vi "UI.vi"(8 "error in (no error)":errorcluster, 10 "subPanel":refnum<vi>, 11 "UI in":refnum<class "UI.lvclass">) -> (0 "error out":errorcluster, 3 "UI out":refnum<class "UI.lvclass">)   [LabVIEW 2019, in "UI.lvclass"]
doc: "Opens the UI Session. You need to pass a SubPanel Reference in order to make your embedded VIs show in it. This is the very first fuction you need to call."
uses:
  UI.lvclass
  UI.lvclass/UI.ctl
  setsubPanel.vi
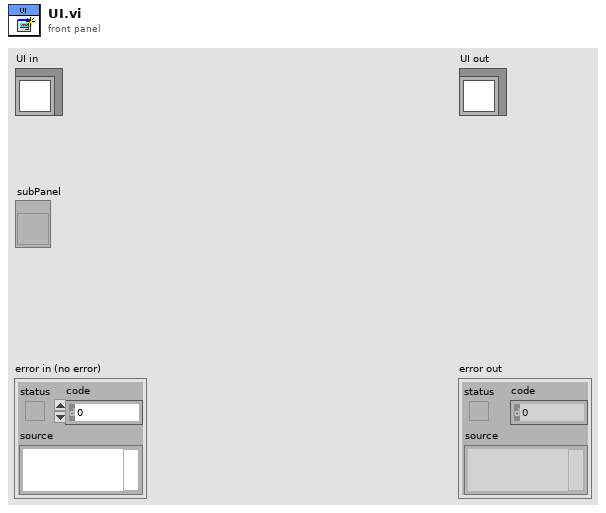
[diagram p1: front panel]
types:
  T1 = enum16{"Create", "Register", "Generate", "Unregister", "Destroy"}
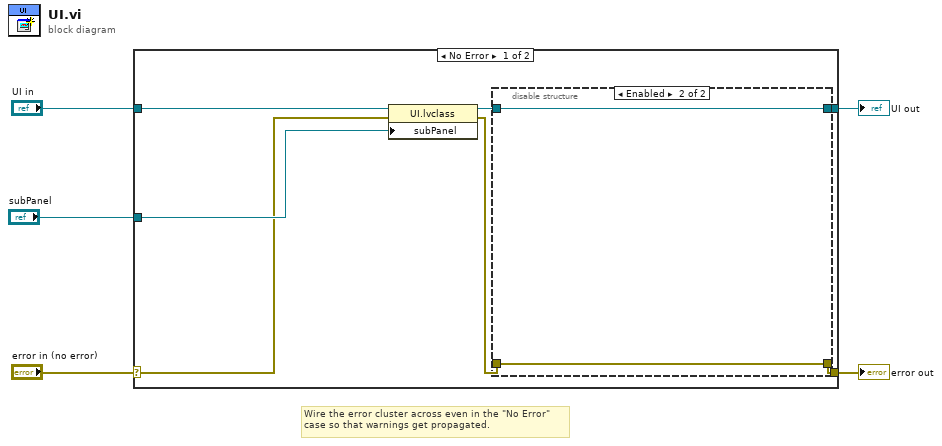
[diagram p0: block diagram]
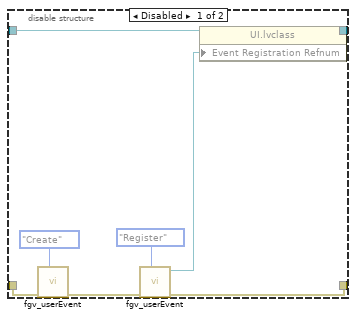
[diagram p2: hidden frame]
diagram:
  # "Wire the error cluster across even in the \"No Error\"\ncase so that warnings get propagated."
  n1 = case shown="No Error" "error in (no error)" {
    selector: "error in (no error)" -> [w9 w24]
    tunnel: [w7 w24] -> w4
    tunnel: [w6 w23] -> w2
    tunnel: "UI in" -> [w12 w23]
    tunnel: "subPanel" -> [w10 _]
    frame No Error {
      n2 = property class="UI.lvclass"(reference=w12, error in=w9, "subPanel"=w10) -> (reference out=w11:refnum<class "UI.lvclass">, error out=w8:errorcluster)
      n3 = disable-structure shown="Enabled" {
        disable-tunnel: w11 -> [w20 w22]
        disable-tunnel: w8 -> [w18 w21]
        disable-tunnel: [w16 w21] -> w7
        disable-tunnel: [w14 w22] -> w6
        frame Disabled {
          n4 = call "fgv_userEvent.vi"("Option"=T1."Create", "Error In"=w18) -> ("Error Out"=w19:errorcluster)  [unwired: 8 in, 1 out]
          n5 = call "fgv_userEvent.vi"("Option"=T1."Register", "Error In"=w19) -> ("Error Out"=w16:errorcluster, "Event Registration Refnum"=w13:refnum<event-registration>)  [unwired: 8 in]
          n6 = property class="UI.lvclass"(reference=w20, "Event Registration Refnum"=w13) -> (reference out=w14:refnum<class "UI.lvclass">)  [unwired: 1 in, 1 out]
        }
        frame Enabled {
        }
      }
    }
    frame Error {
    }
  }
  "error out" <- w4
  "UI out" <- w2
